vi "Save Config.vi"(8 "error in (no error)":errorcluster, 11 "System Config Module in":refnum<class "System Config Module.lvclass">) -> (0 "error out":errorcluster, 3 "System Config Module out":refnum<class "System Config Module.lvclass">)   [LabVIEW 2020, in "Volatus.lvlib" / "System Config Module.lvclass"]
uses:
  System Config Module.lvclass
  System Config Module.lvclass/System Config Module.ctl
  Module/Module.lvclass
  VolatusAPI/VolatusAPI.lvclass
  VolatusConfig/VolatusConfig/VolatusConfig.lvclass
  VolatusConfig/Config Format.ctl
  VolatusConfig/VolatusConfig.lvlib
  C:/dev/lv20CE/relink/lv-volatus/Volatus/Module/Module.lvclass
  C:/dev/lv20CE/relink/lv-volatus/Volatus/System Config Server/System Config Module.lvclass
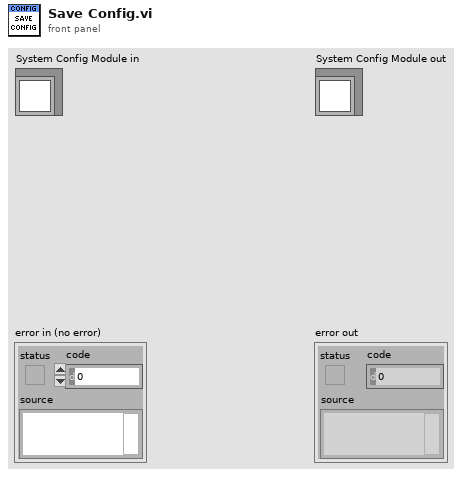
[diagram p1: front panel]
types:
  T1 = typedef "VolatusConfig.lvlib/Config Format.ctl" = enum16{"JSON", "INI", "SQLite"}
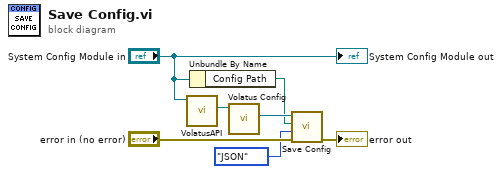
[diagram p0: block diagram]
diagram:
  n1 = call "VolatusAPI.vi"("Module in"="System Config Module in") -> ("VolatusAPI"=w5:refnum<class "VolatusAPI.lvclass">)  [unwired: 9 in, 1 out]
  n2 = Unbundle By Name("System Config Module in") -> ("Config Path"=w3:path)
  n3 = call "Volatus Config.vi"("VolatusAPI in"=w5) -> ("Volatus Config"=w4:refnum<class "VolatusConfig.lvclass">)  [unwired: 8 in, 2 out]
  n4 = call "Save Config.vi"("error in (no error)"="error in (no error)", "Config Format"=Config_Format."JSON", "Path"=w3, "VolatusConfig in"=w4) -> ("error out"=→"error out":errorcluster)  [unwired: 6 in, 1 out]
  "System Config Module out" <- "System Config Module in"
